vi "LVPortUpdateBoundControl.vi"(9 "Controls To Update":refnum<vi>[](array[refnum]), 10 "Control To Update":refnum<vi>, 11 "pID":string) -> (3 "pID out":string)   [LabVIEW 2017]
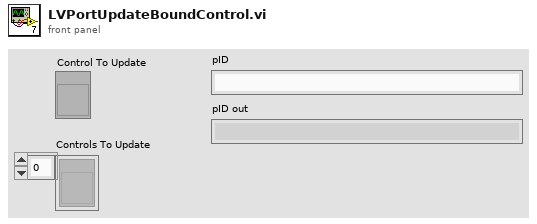
[diagram p1: front panel]
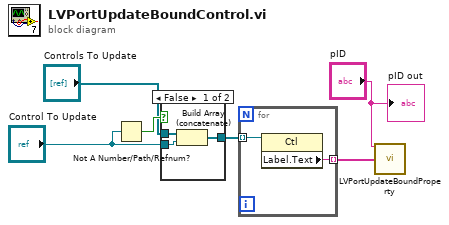
[diagram p0: block diagram]
diagram:
  n1 = Not A Number/Path/Refnum?(number/path/refnum="Control To Update") -> (NaN/Path/Refnum?=w6:bool)
  n2 = case shown="False" w6 {
    tunnel: "Controls To Update" -> [w9 w10]
    tunnel: [w7 w10] -> w2
    tunnel: "Control To Update" -> [w8 _]
    frame False {
      n3 = Build Array (concatenate)(w9, w8) -> (w7:refnum<vi>[])
    }
    frame True {
    }
  }
  n4 = for {
    tunnel: w2 -> [w12] mode=indexing
    tunnel: [w11] -> w1 mode=indexing
    n5 = property class="Ctl"(reference=w12) -> ("Label.Text"=w11:string)  [unwired: 1 in, 2 out]
  }
  n6 = call "LVPortUpdateBoundProperty.vi"("pID"="pID", "Properties"=w1) -> ()  [unwired: 14 in]
  "pID out" <- "pID"
